vi "Detect Modules.vi"(8 "error in":errorcluster, 10 "PXI Module in":refnum<class "PXI Module.lvclass">, 11 "Chassis in":refnum<class "Chassis.lvclass">) -> (0 "error out":errorcluster, 2 "PXI Module out":refnum<class "PXI Module.lvclass">, 3 "Chassis out":refnum<class "Chassis.lvclass">)   [LabVIEW 2016, in "SMI.lvlib" / "PXI Module.lvclass"]
uses:
  PXI Module.lvclass
  Chassis/Chassis.lvclass
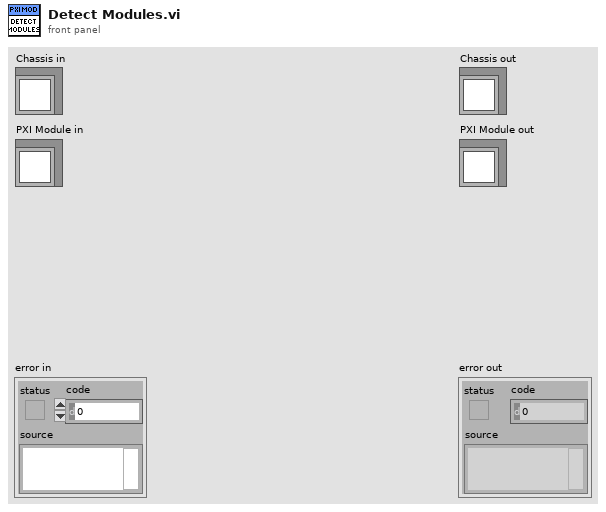
[diagram p1: front panel]
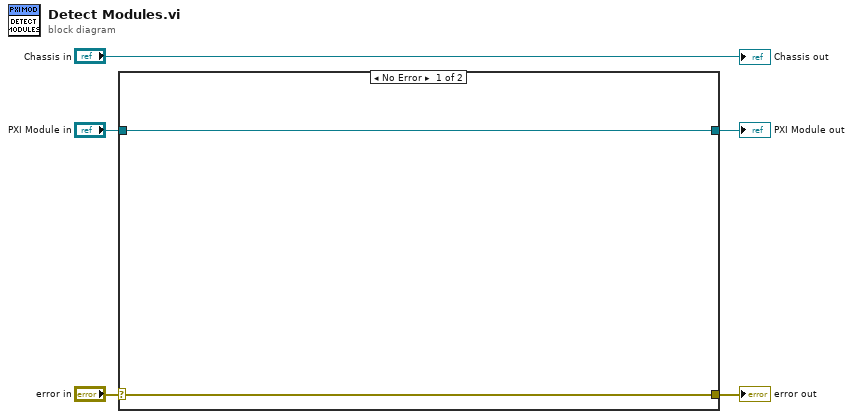
[diagram p0: block diagram]
diagram:
  n1 = case shown="No Error" "error in" {
    selector: "error in" -> [w6 w9]
    tunnel: [w6 w9] -> w4
    tunnel: [w7 w8] -> w2
    tunnel: "PXI Module in" -> [w7 w8]
    frame No Error {
    }
    frame Error {
    }
  }
  "error out" <- w4
  "PXI Module out" <- w2
  "Chassis out" <- "Chassis in"
